vi "SerialCom Initialize_v2.vi"(8 "error in (no error)":errorcluster, 11 "ControlBoard VISA":refnum<visa-resource-name>) -> (0 "error out":errorcluster, 3 "ControlBoard VISA Out":refnum<visa-resource-name>)   [LabVIEW 2022 SP3]
doc: "This VI opens a ControlBoard VISA session and output the VISA reference"
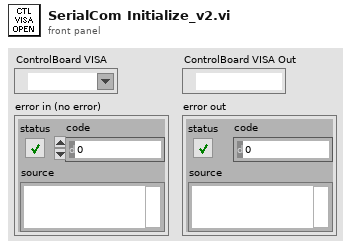
[diagram p1: front panel]
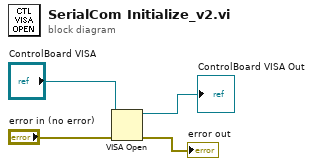
[diagram p0: block diagram]
diagram:
  n1 = VISA Open(error in (no error)="error in (no error)", VISA resource name="ControlBoard VISA") -> (VISA resource name=→"ControlBoard VISA Out":refnum<visa-resource-name>, error out=→"error out":errorcluster)  [unwired: 3 in]
